vi "Cursor List Read.vi"(4 "error in (no error)":errorcluster, 6 "Container State":T3, 7 "Display State In":T1) -> (0 "error out":errorcluster, 2 "Value":T4, 3 "Display State Out":T1)   [LabVIEW 2020, in "3D Waterfall.xctl"]
uses:
  <vilib>/Math Plots/3D Math Plots/3D Waterfall/3D Waterfall XCtrl/3D Waterfall.xctl
  <vilib>/_xctls/Container State.ctl
  <vilib>/Math Plots/3D Math Plots/3D Plot/3D Plot/Typedef/Cursor Property Array.ctl
  <vilib>/Math Plots/3D Math Plots/3D Plot/3D Plot/Typedef/Cursor Property.ctl
  <vilib>/Math Plots/3D Math Plots/3D Plot/3D Plot/Typedef/Cursor Position.ctl
  <vilib>/Math Plots/3D Math Plots/3D Plot/3D Plot/Typedef/Cursor Point.ctl
  <vilib>/Math Plots/3D Math Plots/3D Plot/3D Plot/Typedef/Sprite Type.ctl
  <vilib>/Math Plots/3D Math Plots/3D Plot/3D Plot/Typedef/Cursor Line.ctl
  <vilib>/Math Plots/3D Math Plots/3D Plot/3D Plot/Typedef/Line Type.ctl
  <vilib>/Math Plots/3D Math Plots/3D Plot/3D Plot/Typedef/Cursor Plane.ctl
  <vilib>/Math Plots/3D Math Plots/3D Plot/3D Plot/Typedef/Cursor Text.ctl
  <vilib>/Math Plots/3D Math Plots/3D Waterfall/3D Waterfall XCtrl/State.ctl
  <vilib>/Math Plots/3D Math Plots/3D Waterfall/3D Waterfall/3D Waterfall.lvclass
  e:/builds/penguin/labview/branches/2020/dev/dist/vi.lib/Math Plots/3D Math Plots/3D Plot/3D Plot/3D Plot.lvclass
  <vilib>/Math Plots/3D Math Plots/3D Plot/Action String/3DMathPlot Ctrl Act Queue.ctl
  <vilib>/Math Plots/3D Math Plots/3D Plot/Action String/3DMathPlot Ctrl Act Cluster.ctl
  <vilib>/Math Plots/3D Math Plots/3D Plot/Action String/3DMathPlot State Class.ctl
  <vilib>/Math Plots/3D Math Plots/3D Plot/3D Plot/3D Plot.lvclass
  <vilib>/_xctls/XControlSupport.lvlib
panel:
  # "Replace the Value Indicator below with an Indicator of desired type.\nDo not remove this Indicator or the others from the connector pane. \nDo not change the connector pane pattern.\nThe Value Indicator should always be the second terminal from top on the output side in the connector pane."
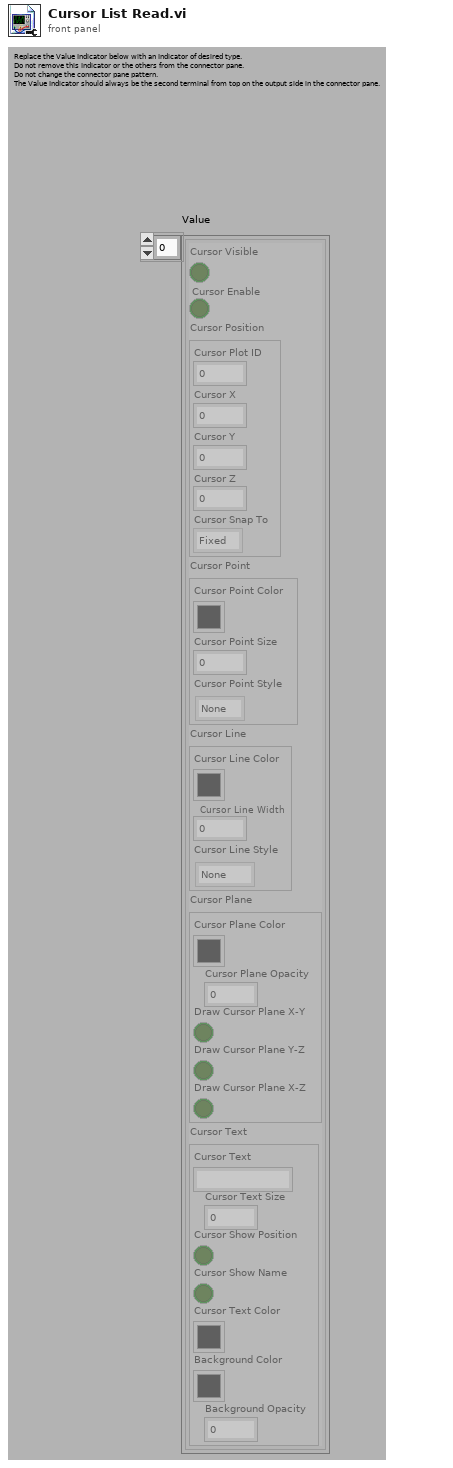
[diagram p1: front panel]
types:
  T1 = typedef "3D Waterfall.xctl/State.ctl" = cluster{"3D Waterfall.lvclass":refnum<class "3D Waterfall.lvclass">, "Control Ref Queue":T2, "Main Frame Color":u32, "Ramp Palette Color":u32, "Projection Palette Color":u32}
  T2 = typedef "3DMathPlot Ctrl Act Queue.ctl" = refnum<queue>
  T3 = typedef "XControlSupport.lvlib/Container State.ctl" = cluster{"Indicator?":bool, "Run Mode?":bool, " Refnum":refnum<vi>}
  T4 = typedef "3D Plot.lvclass/Cursor Property Array.ctl" = T5[]
  T5 = typedef "3D Plot.lvclass/Cursor Property.ctl" = cluster{"Cursor Visible":bool, "Cursor Enable":bool, "Cursor Position":T6, "Cursor Point":T7, "Cursor Line":T9, "Cursor Plane":T11, "Cursor Text":T12}
  T6 = typedef "3D Plot.lvclass/Cursor Position.ctl" = cluster{"Cursor Plot ID":i32, "Cursor X":sgl, "Cursor Y":sgl, "Cursor Z":sgl, "Cursor Snap To":enum16{"Fixed", "Nearest Plot", "Snap to Plot"}}
  T7 = typedef "3D Plot.lvclass/Cursor Point.ctl" = cluster{"Cursor Point Color":u32, "Cursor Point Size":sgl, "Cursor Point Style":T8}
  T8 = typedef "3D Plot.lvclass/Sprite Type.ctl" = enum16{"None", "Empty Square", "Solid Square", "Empty Diamond", "Solid Diamond", "Empty Circle", "Solid Circle", "Asterisk", "Bold X", "Wireframe Sphere", "Solid Sphere", "Wireframe Cube", "Solid Cube"}
  T9 = typedef "3D Plot.lvclass/Cursor Line.ctl" = cluster{"Cursor Line Color":u32, "Cursor Line Width":sgl, "Cursor Line Style":T10}
  T10 = typedef "3D Plot.lvclass/Line Type.ctl" = enum16{"None", "Solid", "Dash", "Dot", "Dash Dot"}
  T11 = typedef "3D Plot.lvclass/Cursor Plane.ctl" = cluster{"Cursor Plane Color":u32, "Cursor Plane Opacity":sgl, "Draw Cursor Plane X-Z":bool, "Draw Cursor Plane Y-Z":bool, "Draw Cursor Plane X-Y":bool}
  T12 = typedef "3D Plot.lvclass/Cursor Text.ctl" = cluster{"Cursor Text":string, "Cursor Text Size":u16, "Cursor Show Position":bool, "Cursor Show Name":bool, "Cursor Text Color":u32, "Background Color":u32, "Background Opacity":sgl}
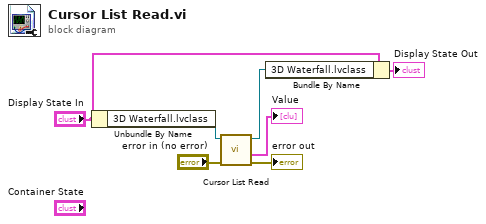
[diagram p0: block diagram]
diagram:
  n1 = Unbundle By Name("Display State In") -> ("3D Waterfall.lvclass"=w7:refnum<class "3D Waterfall.lvclass">)
  n2 = call <vilib>:"Cursor List Read.vi"("error in (no error)"="error in (no error)", "3D Plot.lvclass in"=w7) -> ("error out"=→"error out":errorcluster, "Cursor Property Array"=→"Value":T4, "3D Plot.lvclass out"=w6:refnum<class "3D Waterfall.lvclass">)  [unwired: 7 out]
  n3 = Bundle By Name(cluster="Display State In", "3D Waterfall.lvclass"=w6) -> (→"Display State Out":T1)
